vi "Read Scalar DBL.vi"(8 "error in (no error)":errorcluster, 11 "pointer in":u64) -> (0 "error out":errorcluster, 2 "value out":dbl, 3 "pointer out":u64)   [LabVIEW 2013, in "Linux RT IPC.Shared Memory.lvlib"]
uses:
  Linux RT IPC.Shared Memory.lvlib
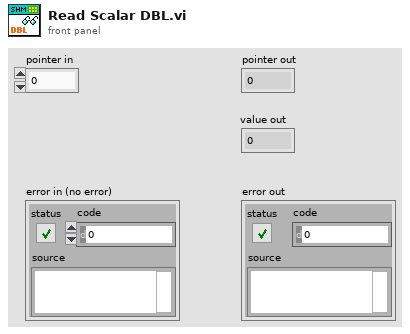
[diagram p1: front panel]
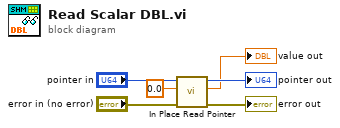
[diagram p0: block diagram]
diagram:
  n1 = call-poly "In Place Read Pointer.vi"("error in (no error)"="error in (no error)", "value in"=0.0, "pointer in"="pointer in") -> ("error out"=→"error out":errorcluster, "value out"=→"value out":dbl, "pointer out"=→"pointer out":u64)  [unwired: 6 in]
